vi "11.15-Single-SideFFT.vi"() -> ()   [LabVIEW 2018]
uses:
  <vilib>/Analysis/2dsp.llb/Real FFT.vi
  <vilib>/Analysis/NI_AALPro.lvlib
  <vilib>/Analysis/NI_AALBase.lvlib
panel:
  in  "停止":bool
  out "频谱索引":i32[](array[numeric])
  out "最大幅值":dbl
  in  "FFT size":i32=-1 caption="FFT点数"
  in  "shift?":bool caption="移位？"
  out "单边FFT变换":cluster{dbl, dbl, dbl[]}(graph)
  out "信号波形":cluster{dbl[unit], dbl[unit], "sine wave":dbl[]}(graph)
  in  "采样频率":dbl=100.0
  in  "frequency":dbl=5.0 caption="频率(Hz)" format="%.4f"
  in  "amplitude":dbl=1.0 caption="幅值" format="%0.2f"
  in  "采样点数":i32=100
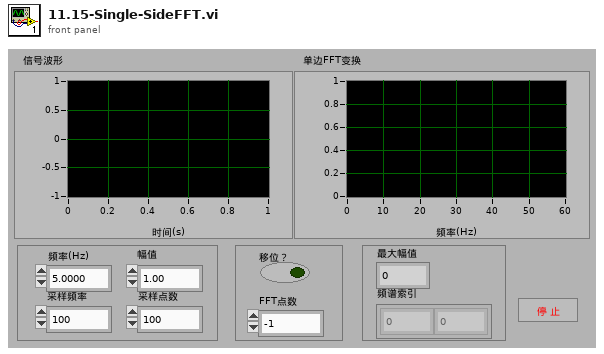
[diagram p1: front panel]
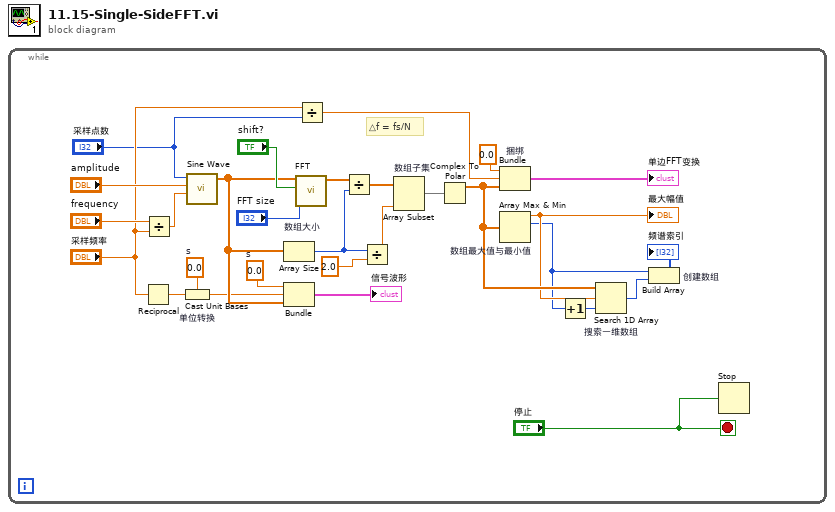
[diagram p0: block diagram]
diagram:
  n1 = while {
    stop <- "停止" stop-if-true
    w11 = dbl[unit] 0.0  # s
    w14 = dbl[unit] 0.0  # s
    # "△f = fs/N"
    n2 = Reciprocal(x="采样频率") -> (1/x=w10:dbl)
    n3 = Divide(x="frequency", y="采样频率") -> (x/y=w27:dbl)
    n4 = Cast Unit Bases "单位转换"(0:w10, 1:w11) -> (2:w12:dbl[unit])
    n5 = call <vilib>:"Sine Wave.vi"("samples"="采样点数", "amplitude"="amplitude", "frequency"=w27) -> ("sine wave"=w13:dbl[])  [unwired: 2 in, 2 out]
    n6 = Array Size "数组大小"(array=w13) -> (size(s)=w6:i32)
    n7 = Bundle(w14, w12, "sine wave"=w13) -> (→"信号波形":cluster{dbl[unit], dbl[unit], "sine wave":dbl[]})  [unwired: 1 in]
    n8 = call-poly <vilib>:"FFT.vi"("FFT size"="FFT size", "shift?"="shift?", "X"=w13) -> ("FFT {X}"=w24:cdb[])  [unwired: 7 in, 1 out]
    n9 = Divide(x="采样频率", y="采样点数") -> (x/y=w4:dbl)
    n10 = Divide(x=w24, y=w6) -> (x/y=w9:cdb[])
    n11 = Divide(x=w6, y=2.0) -> (x/y=w7:dbl)
    n12 = Array Subset "数组子集"(array=w9, length=w7) -> (w8:cdb[])  [unwired: 1 in]
    n13 = Complex To Polar(r * e^(i*theta)=w8) -> (r=w21:dbl[])  [unwired: 1 out]
    n14 = Bundle "捆绑"(0.0, w4, w21) -> (→"单边FFT变换":cluster{dbl, dbl, dbl[]})  [unwired: 1 in]
    n15 = Array Max & Min "数组最大值与最小值"(array=w21) -> (max value=w20:dbl, max index (indices)=w18:i32)  [unwired: 2 out]
    "最大幅值" <- w20
    n16 = Increment(x=w18) -> (x+1=w19:i32)
    n17 = Search 1D Array "搜索一维数组"(1D array=w21, element=w20, start index (0)=w19) -> (index of element=w17:i32)
    n18 = Build Array "创建数组"(w18, w17) -> (→"频谱索引":i32[])
    n19 = Stop(stop? (T)="停止") -> ()
  }
